vi "Init_stim_tasks_NI.vi"(6 "error in":errorcluster, 8 "Run mode":T1, 9 "Device parameters":T2={"Triggered?"=FALSE, "Shutter channel"="", "Acquisition channels"="", "Acquisition sample rate"=0.0, "Read chunk size"=0, "Stimulation channel"="Dev1/ao0", "Stimulation sample rate"=0.0} {"Read chunk size" min=100 max=100000; "Acquisition sample rate" min=10.0 max=10000.0 step=10.0; "Stimulation sample rate" min=10.0 max=10000.0}) -> (0 "error out":errorcluster, 3 "Stim task out":refnum<k21>)   [LabVIEW 2011]
uses:
  typedefs/device_parameters.ctl
  typedefs/run_mode.ctl
  <vilib>/DAQmx/create/channels.llb/DAQmx Create Channel (AO-Voltage-Basic).vi
  <vilib>/DAQmx/configure/timing.llb/DAQmx Timing (Sample Clock).vi
  <vilib>/DAQmx/configure/trigger.llb/DAQmx Start Trigger (Digital Edge).vi
  Program Files/National Instruments/LabVIEW 2011/resource/objmgr/daqmx.rc
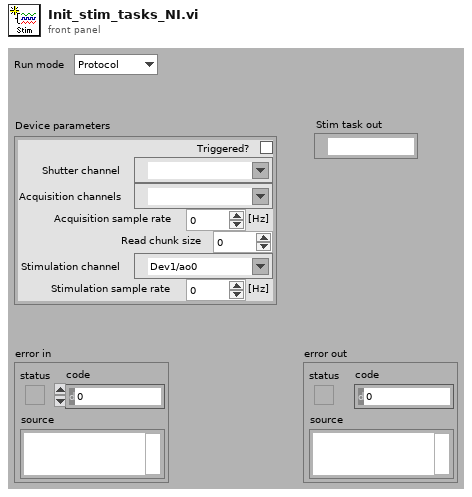
[diagram p1: front panel]
types:
  T1 = typedef "run_mode.ctl" = enum32{"Protocol", "Free Run"}
  T2 = typedef "device_parameters.ctl" = cluster{"Triggered?":bool, "Shutter channel":tag, "Acquisition channels":tag, "Acquisition sample rate":dbl, "Read chunk size":i32, "Stimulation channel":tag, "Stimulation sample rate":dbl}
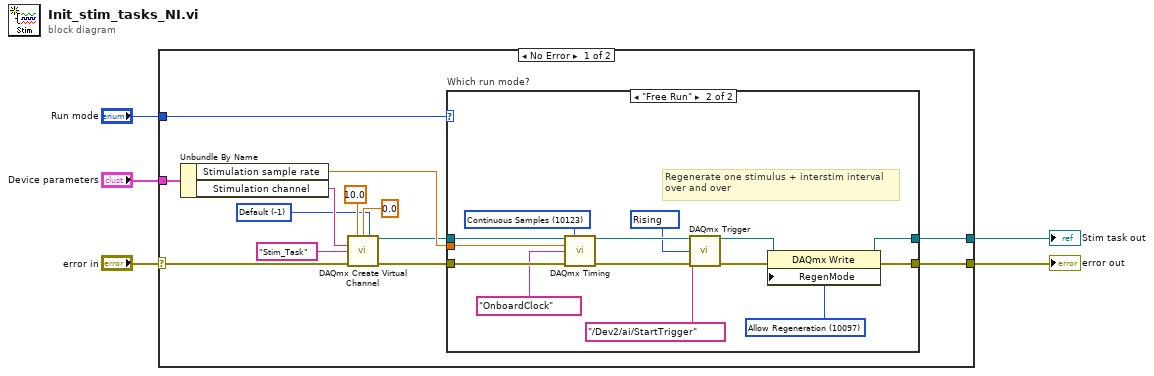
[diagram p0: block diagram]
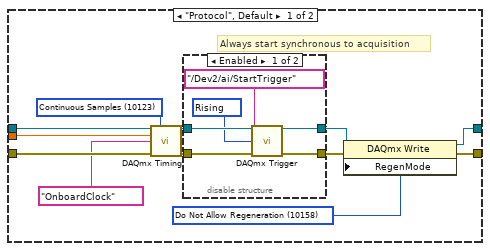
[diagram p2: hidden frame]
diagram:
  n1 = case shown="No Error" "error in" {
    selector: "error in" -> [w9 w53]
    tunnel: [w8 w53] -> w5
    tunnel: "Device parameters" -> [w10 _]
    tunnel: [w11 _] -> w3
    tunnel: "Run mode" -> [w7 _]
    frame No Error {
      w6 = -1 items=["Default"=-1, "RSE"=10083, "Differential"=10106, "Pseudodifferential"=12529] ("output terminal configuration")
      n2 = Unbundle By Name(w10) -> ("Stimulation sample rate"=w18:dbl, "Stimulation channel"=w16:tag)
      n3 = call-poly <vilib>:"DAQmx Create Virtual Channel.vi"("maximum value"=10.0, "minimum value"=0.0, "output terminal configuration"=w6, "physical channels"=w16, "name to assign"="Stim_Task", "error in"=w9) -> ("task out"=w12:refnum<k21>, "error out"=w17:errorcluster)  [unwired: 8 in]
      n4 = case "Which run mode?" shown="\"Free Run\"" w7 {
        tunnel: w18 -> [w28 w50]
        tunnel: w17 -> [w27 w49]
        tunnel: w12 -> [w26 w48]
        tunnel: [w21 w40] -> w11
        tunnel: [w20 w41] -> w8
        frame "Protocol", Default {
          w19 = 10158 items=["Allow Regeneration"=10097, "Do Not Allow Regeneration"=10158] ("RegenMode")
          w24 = 10123 items=["Finite Samples"=10178, "Continuous Samples"=10123, "Hardware Timed Single Point"=12522] ("sample mode")
          # "Always start synchronous to acquisition"
          n5 = call-poly <vilib>:"DAQmx Timing.vi"("task/channels in"=w26, "sample mode"=w24, "rate"=w28, "source"=tag "OnboardClock", "error in"=w27) -> ("task out"=w30:refnum<k21>, "error out"=w29:errorcluster)  [unwired: 9 in]
          n6 = disable-structure shown="Enabled" {
            disable-tunnel: w30 -> [w36 w38]
            disable-tunnel: w29 -> [w35 w37]
            disable-tunnel: [w32 w37] -> w23
            disable-tunnel: [w31 w38] -> w22
            frame Enabled {
              w33 = 10280 items=["Rising"=10280, "Falling"=10171] ("edge")
              n7 = call-poly <vilib>:"DAQmx Trigger.vi"("task/channels in"=w36, "source"=tag "/Dev2/ai/StartTrigger", "edge"=w33, "error in"=w35) -> ("task out"=w31:refnum<k21>, "error out"=w32:errorcluster)  [unwired: 10 in]
            }
            frame Disabled {
            }
          }
          n8 = property class="DAQmx Write"(reference=w22, error in=w23, "RegenMode"=w19) -> (reference out=w21:refnum<k21>, error out=w20:errorcluster)
        }
        frame "Free Run" {
          w39 = 10097 items=["Allow Regeneration"=10097, "Do Not Allow Regeneration"=10158] ("RegenMode")
          w44 = 10280 items=["Rising"=10280, "Falling"=10171] ("edge")
          w46 = 10123 items=["Finite Samples"=10178, "Continuous Samples"=10123, "Hardware Timed Single Point"=12522] ("sample mode")
          # "Regenerate one stimulus + interstim interval\nover and over"
          n9 = call-poly <vilib>:"DAQmx Timing.vi"("task/channels in"=w48, "sample mode"=w46, "rate"=w50, "source"=tag "OnboardClock", "error in"=w49) -> ("task out"=w52:refnum<k21>, "error out"=w51:errorcluster)  [unwired: 9 in]
          n10 = call-poly <vilib>:"DAQmx Trigger.vi"("task/channels in"=w52, "source"=tag "/Dev2/ai/StartTrigger", "edge"=w44, "error in"=w51) -> ("task out"=w43:refnum<k21>, "error out"=w42:errorcluster)  [unwired: 10 in]
          n11 = property class="DAQmx Write"(reference=w43, error in=w42, "RegenMode"=w39) -> (reference out=w40:refnum<k21>, error out=w41:errorcluster)
        }
      }
    }
    frame Error {
    }
  }
  "error out" <- w5
  "Stim task out" <- w3
